vi "test-linear-filter-test-03-derivA.vi"(11 "Input":dbl) -> (3 "Output":dbl)   [LabVIEW 2019]
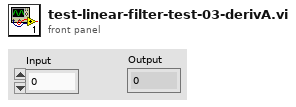
[diagram p1: front panel]
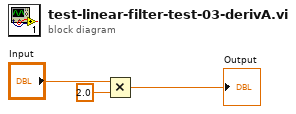
[diagram p0: block diagram]
diagram:
  n1 = Multiply(x="Input", y=2.0) -> (x*y=→"Output":dbl)
